vi "AlliGator Is IRF Valid.vi"(2 "Reference Decay":cluster{"t Array":dbl[], "I Array":dbl[]}) -> (7 "Valid Plot?":bool)   [LabVIEW 2021, in "AlliGator IRF.lvlib"]
doc: "Checks that the <B>Reference Decay</B> is a valid plot."
uses:
  AlliGator IRF.lvlib
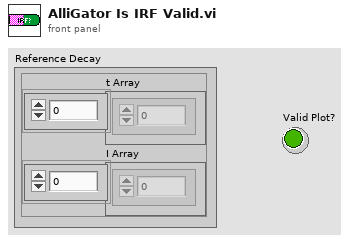
[diagram p1: front panel]
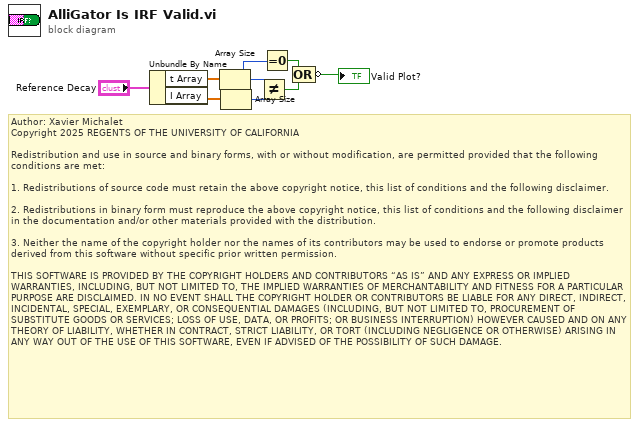
[diagram p0: block diagram]
diagram:
  # "Author: Xavier Michalet\nCopyright 2025 REGENTS OF THE UNIVERSITY OF CALIFORNIA\n\nRedistribution and use in source and binary forms, with or without modification, are permitted provided that the following conditions are met:\n\n1. Redistributions of source code must retain the above copyright notice, this list of conditions and the following disclaimer.\n\n2. Redistributions in binary form must reproduce the above copyright notice, this list of conditions and the following disclaimer in the documentation and/or other materials provided with the distribution.\n\n3. Neither the name of the copyright holder nor the names of its contributors may be used to endorse or promote products derived from this software without specific prior written permission.\n\nTHIS SOFTWARE IS PROVIDED BY THE COPYRIGHT HOLDERS AND CONTRIBUTORS “AS IS” AND ANY EXPRESS OR IMPLIED WARRANTIES, INCLUDING, BUT NOT LIMITED TO, THE IMPLIED WARRANTIES OF MERCHANTABILITY AND FITNESS FOR A PARTICULAR PURPOSE ARE DISCLAIMED. IN NO EVENT SHALL THE COPYRIGHT HOLDER OR CONTRIBUTORS BE LIABLE FOR ANY DIRECT, INDIRECT, INCIDENTAL, SPECIAL, EXEMPLARY, OR CONSEQUENTIAL DAMAGES (INCLUDING, BUT NOT LIMITED TO, PROCUREMENT OF SUBSTITUTE GOODS OR SERVICES; LOSS OF USE, DATA, OR PROFITS; OR BUSINESS INTERRUPTION) HOWEVER CAUSED AND ON ANY THEORY OF LIABILITY, WHETHER IN CONTRACT, STRICT LIABILITY, OR TORT (INCLUDING NEGLIGENCE OR OTHERWISE) ARISING IN ANY WAY OUT OF THE USE OF THIS SOFTWARE, EVEN IF ADVISED OF THE POSSIBILITY OF SUCH DAMAGE."
  n1 = Unbundle By Name("Reference Decay") -> ("t Array"=w7:dbl[], "I Array"=w6:dbl[])
  n2 = Array Size(array=w7) -> (size(s)=w4:i32)
  n3 = Array Size(array=w6) -> (size(s)=w5:i32)
  n4 = Not Equal?(x=w4, y=w5) -> (x != y?=w2:bool)
  n5 = Equal To 0?(x=w4) -> (x = 0?=w3:bool)
  n6 = Compound Arithmetic op=OR(w3, w2) -> (invert →"Valid Plot?":bool)
